vi "Loop_CalculateDegree (SubVI).vi"(9 "Desired Degree":dbl, 11 "Max Encoder Ticks (1 Rotation)":dbl format="%#_13g") -> (3 "Output Position":dbl)   [LabVIEW 2017]
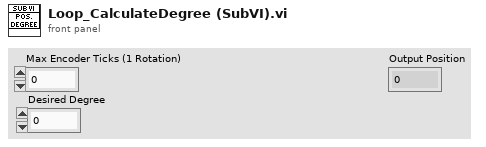
[diagram p1: front panel]
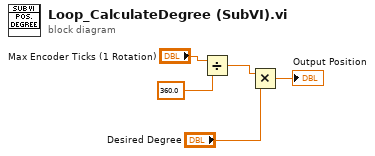
[diagram p0: block diagram]
diagram:
  n1 = Divide(x="Max Encoder Ticks (1 Rotation)", y=360.0) -> (x/y=w3:dbl)
  n2 = Multiply(x=w3, y="Desired Degree") -> (x*y=→"Output Position":dbl)
